vi "finishGoalKickAllyPlayVSS.vi"(8 "error in (no error)":errorcluster, 10 "Game in":refnum<class "Game.lvclass">, 11 "GoalKickAllyPlayVSS in":refnum<class "GoalKickAllyPlayVSS.lvclass">) -> (0 "error out":errorcluster, 2 "result":bool, 3 "GoalKickAllyPlayVSS out":refnum<class "GoalKickAllyPlayVSS.lvclass">)   [LabVIEW 2023, in "GoalKickAllyPlayVSS.lvclass"]
uses:
  GoalKickAllyPlayVSS.lvclass
  Game_class/Game.lvclass
  Game_class/Game.lvclass/Game.ctl
  Events_class/Events.lvclass/Events.ctl
  Game_class/Read Referee.vi
  Game_class/Read EventsRef.vi
  Events_class/Read id_touch.vi
  Referee_class/Referee.lvclass
  Events_class/Events.lvclass
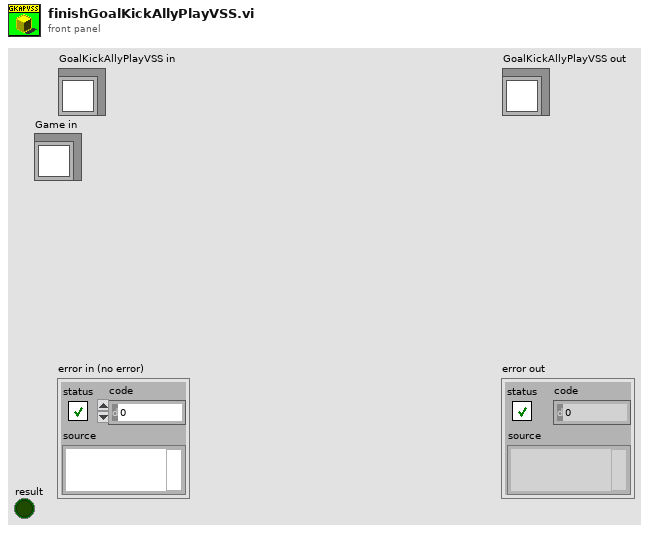
[diagram p1: front panel]
types:
  T1 = enum16{"AUTO", "GAME_ON", "STOP", "KICKOFF", "FREE_BALL", "GOAL_KICK", "PENALTY_KICK", "FREE_KICK"}
  T2 = typedef "Command.ctl" = enum16{"AUTO", "GAME_ON", "STOP", "HALT", "KICKOFF_ALLY", "KICKOFF_ENEMY", "FREE_BALL", "GOAL_KICK_ENEMY", "GOAL_KICK_ALLY", "PENALTY_KICK_ENEMY", "PENALTY_KICK_ALLY", "FREE_KICK"}
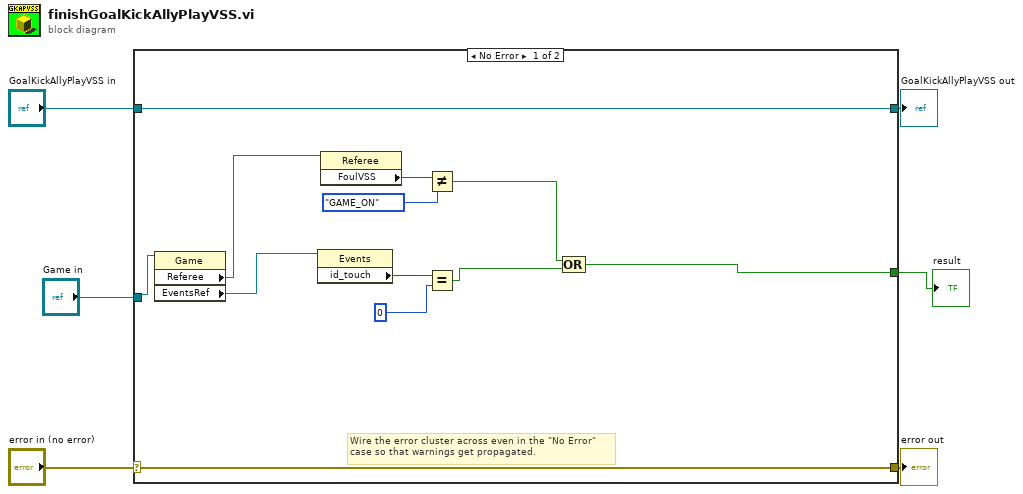
[diagram p0: block diagram]
diagram:
  n1 = case shown="No Error" "error in (no error)" {
    selector: "error in (no error)" -> [w17 w20]
    tunnel: [w17 w20] -> w5
    tunnel: [w18 w19] -> w3
    tunnel: "GoalKickAllyPlayVSS in" -> [w18 w19]
    tunnel: "Game in" -> [w15 _]
    tunnel: [w14 _] -> w1
    frame No Error {
      # "Wire the error cluster across even in the \"No Error\"\ncase so that warnings get propagated."
      n2 = property class="Game"(reference=w15) -> ("Referee"=w11:refnum<class "Referee.lvclass">, "EventsRef"=w16:refnum<class "Events.lvclass">)  [unwired: 1 in, 2 out]
      n3 = property class="Events"(reference=w16) -> ("id_touch"=w8:i32)  [unwired: 1 in, 2 out]
      n4 = property class="Referee"(reference=w11) -> ("FoulVSS"=w13:T2)  [unwired: 1 in, 2 out]
      n5 = Not Equal?(x=w13, y=T1."GAME_ON") -> (x != y?=w10:bool)
      n6 = Equal?(x=w8, y=0) -> (x = y?=w7:bool)
      n7 = Compound Arithmetic op=OR(w10, w7) -> (w14:bool)
    }
    frame Error {
    }
  }
  "error out" <- w5
  "GoalKickAllyPlayVSS out" <- w3
  "result" <- w1
